vi "Create Indices.vi"(8 "error in":errorcluster[](array[cluster]), 11 "connection in":refnum<k13>[](array[refnum])) -> (0 "error out":errorcluster[](array[cluster]), 1 "Indices":i32[](array[numeric]), 2 "Dnet Output Bytes":u8[](array[numeric]), 3 "connection out":refnum<k13>[](array[refnum]))   [LabVIEW 2011]
uses:
  GlobalVariables.vi
panel:
  out "Count":i32
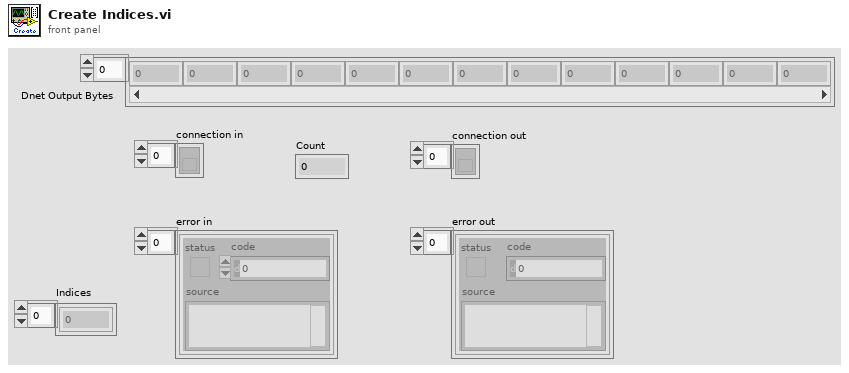
[diagram p1: front panel]
types:
  T1 = typedef "Device Cluster.ctl" = cluster{"Dnet":string, "Node":i32, "Type":string, "ID Number":u8, "SCCM":dbl, "FullScale":dbl, "Input Bytes":i32, "Output Bytes":i32, "Input Start Location":i32, "Output Start Location":i32, "Enabled":bool, "Bytes":u8[]}
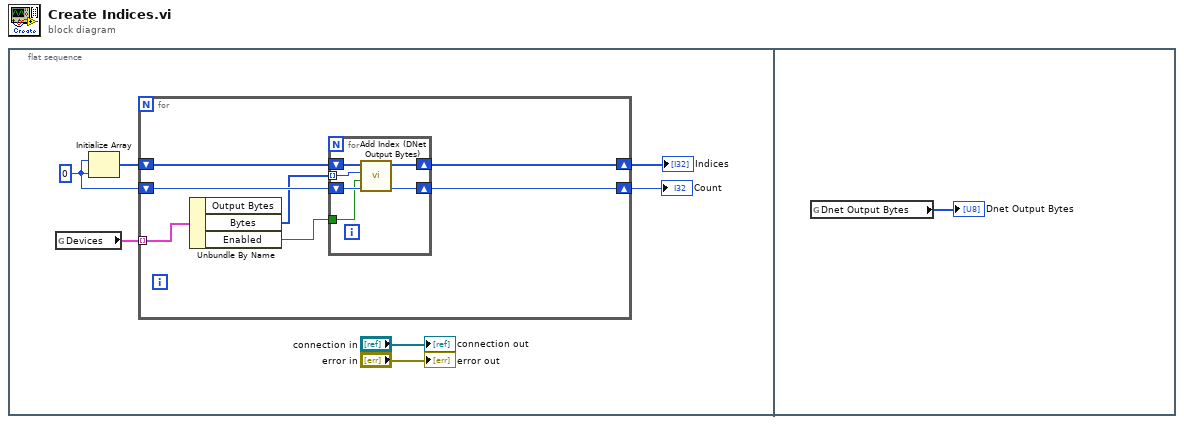
[diagram p0: block diagram]
diagram:
  n1 = flat-sequence {
    frame #0 {
      w1 = 0 ("dimension size")
      n2 = global read "GlobalVariables.vi" "Devices"() -> (w5:T1[])
      n3 = Initialize Array(w1, w1) -> (w3:i32[])
      n4 = for {
        tunnel: w5 -> [w14] mode=indexing
        shift-right: [w12] -> w4
        shift-left: w3 -> [w13]
        shift-right: [w10] -> w2
        shift-left: w1 -> [w11]
        n5 = Unbundle By Name(w14) -> ("Bytes"=w9:u8[], "Enabled"=w8:bool)  [unwired: 1 out]
        n6 = for {
          shift-right: [w19] -> w12
          shift-left: w13 -> [w20]
          shift-right: [w17] -> w10
          shift-left: w11 -> [w18]
          tunnel: w9 -> [w16] mode=indexing
          tunnel: w8 -> [w15]
          n7 = call "Add Index (DNet Output Bytes).vi"("Count"=w18, "Enabled"=w15, "Byte"=w16, "Indices Input"=w20) -> ("Count+1"=w17:i32, "Indices Output"=w19:i32[])  [unwired: 6 in]
        }
      }
      "Indices" <- w4
      "Count" <- w2
      "connection out" <- "connection in"
      "error out" <- "error in"
    }
    frame #1 {
      n8 = global read "GlobalVariables.vi" "Dnet Output Bytes"() -> (→"Dnet Output Bytes":u8[])
    }
  }
